vi "Stream Opts.vi"(8 "error in (no error)":errorcluster, 11 "Websocket Client in":refnum<class "Websocket Client.lvclass">) -> (0 "error out":errorcluster, 3 "Websocket Client out":refnum<class "Websocket Client.lvclass">, 5 "Timeout ms":i32)   [LabVIEW 2020, in "Stream-Websocket.lvlib" / "Websocket Client.lvclass"]
uses:
  Websocket Client.lvclass
  Websocket Client.lvclass/Websocket Client.ctl
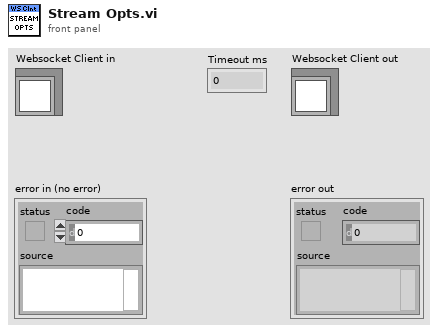
[diagram p1: front panel]
types:
  T1 = typedef "Stream-Websocket.lvlib/Websocket Client.lvclass/Ref Data.ctl" = cluster{"TCP Connection":refnum<k5>, "WS Stream":refnum<class "WebsocketStream.lvclass">, "Connection Loop":refnum<vi>, "Timeout ms":i32, "Server Connection":bool}
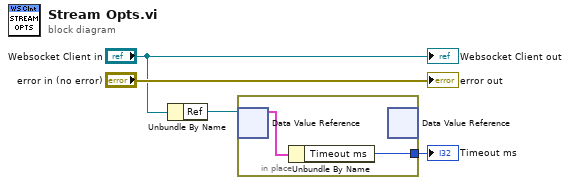
[diagram p0: block diagram]
diagram:
  n1 = Unbundle By Name("Websocket Client in") -> ("Ref"=w3:refnum<data-value>)
  n2 = in-place {
    in-place-border: [w5] -> w1
    n3 = in-place-dvr #1(w3) -> (w6:T1)  [unwired: 1 out]
    n4 = Unbundle By Name(w6) -> ("Timeout ms"=w5:i32)
    n5 = in-place-dvr #1() -> ()  [unwired: 1 in, 2 out]
  }
  "Timeout ms" <- w1
  "error out" <- "error in (no error)"
  "Websocket Client out" <- "Websocket Client in"
